vi "String_to_DataType.vi"(4 "data type string":string) -> (1 "data type":T1)   [LabVIEW 2016, in "PyLVi.lvlib" / "PyLVi.lvclass"]
uses:
  PyLVi.lvclass
  Controls/DataType.ctl
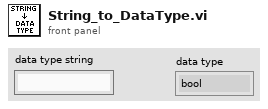
[diagram p1: front panel]
types:
  T1 = typedef "PyLVi.lvlib/PyLVi.lvclass/DataType.ctl" = enum16{"bool", "string", "int16", "int32", "float32", "float64", "complex128"}
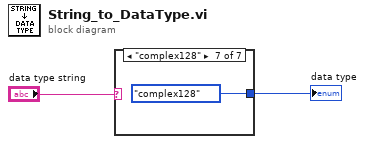
[diagram p0: block diagram]
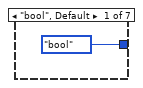
[diagram p2: hidden frame]
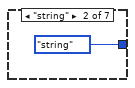
[diagram p3: hidden frame]
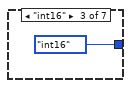
[diagram p4: hidden frame]
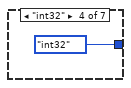
[diagram p5: hidden frame]
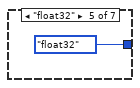
[diagram p6: hidden frame]
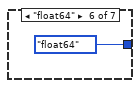
[diagram p7: hidden frame]
diagram:
  n1 = case shown="\"complex128\"" "data type string" {
    tunnel: [DataType."bool" ("data type") DataType."string" ("data type") DataType."int16" ("data type") DataType."int32" ("data type") DataType."float32" ("data type") DataType."float64" ("data type") DataType."complex128" ("data type")] -> w1
    frame "bool", Default {
    }
    frame "string" {
    }
    frame "int16" {
    }
    frame "int32" {
    }
    frame "float32" {
    }
    frame "float64" {
    }
    frame "complex128" {
    }
  }
  "data type" <- w1
